vi "MagBrakeToggle (1).vi"(8 "MagBrake Out":bool, 9 "MagBrake In":bool, 10 "MagPressureLimit (PSI)":dbl, 11 "MagBrakeOn?":bool) -> (1 "MagBrake OUTPUT":bool, 2 "MagBrake In":bool, 3 "MagBrakeToggle Complete":bool)   [LabVIEW 2017]
uses:
  Sensors/DataStreamIndex.ctl
  HostDataGLOBAL.vi
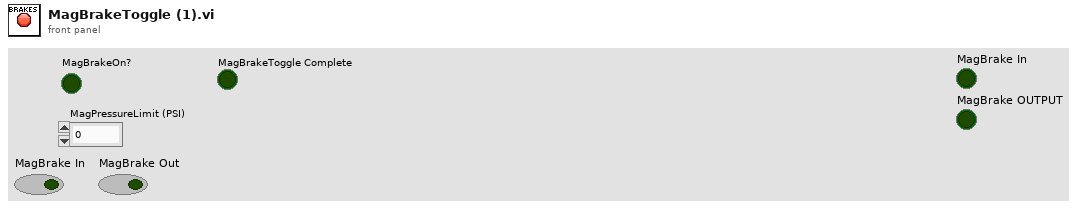
[diagram p1: front panel]
types:
  T1 = typedef "DataStreamIndex.ctl" = enum16{"SuspensionPT (PSI)", "MagBrakePT (PSI)", "Baby HPPT (PSI)", "BigRight HPPT (PSI)", "BigLeft HPPT (PSI)", "HallEffect FrontLeft (V)", "HallEffect FrontRight (V)", "HallEffect BackRight (V)", "HallEffect BackLeft (V)", "LinearPot FrontRight (V)", "LinearPot FrontLeft (V)", "LinearPot BackRight (V)", "LinearPot BackLeft (V)", "Speed (m/s)", "Distance (m)", "Piezo (V)", "Battery Voltage (V)", "Battery Current", "Battery Temperature (C)", "cRIO Temperature (C)", "Right Big Tank Temperature (C)", "Left Big Tank Temperature (C)", "Baby Tank Temperature (C)", "Right Manifold Temperature (C)", "Left Manifold Temperature (C)", "IMU Acceleration (m/s2)", "IMU Pressure (Pa)", "IMU Temperature (C)"}
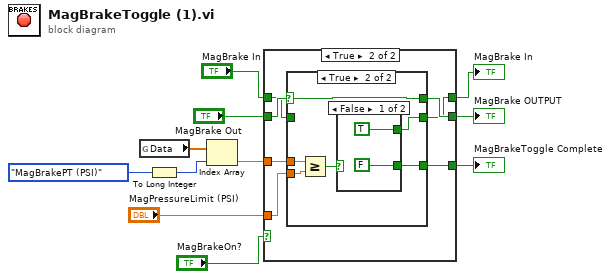
[diagram p0: block diagram]
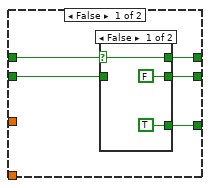
[diagram p2: hidden frame]
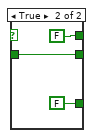
[diagram p3: hidden frame]
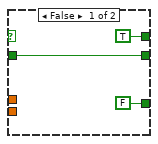
[diagram p4: hidden frame]
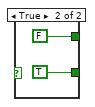
[diagram p5: hidden frame]
diagram:
  n1 = global read "HostDataGLOBAL.vi" "Data"() -> (w4:dbl[])
  n2 = To Long Integer(number=DataStreamIndex."MagBrakePT (PSI)" ("Data Stream Index")) -> (32bit integer=w1:i32)
  n3 = Index Array(array=w4, index=w1) -> (element=w2:dbl)
  n4 = case shown="True" "MagBrakeOn?" {
    tunnel: "MagBrake Out" -> [w13 w29]
    tunnel: [w14 w28] -> w7
    tunnel: [w15 w27] -> w8
    tunnel: "MagBrake In" -> [w16 w26]
    tunnel: "MagPressureLimit (PSI)" -> [_ w25]
    tunnel: w2 -> [_ w24]
    tunnel: [w12 w23] -> w9
    frame False {
      n5 = case shown="False" w16 {
        selector: w16 -> [w18 _]
        tunnel: [w18 FALSE] -> w15
        tunnel: [FALSE ("MagBrake OUTPUT") w21] -> w14
        tunnel: w13 -> [_ w21]
        tunnel: [TRUE FALSE] -> w12
        frame False {
        }
        frame True {
        }
      }
    }
    frame True {
      n6 = case shown="True" w29 {
        selector: w29 -> [_ w38]
        tunnel: [TRUE w38] -> w28
        tunnel: [w31 w36] -> w27
        tunnel: w26 -> [w31 _]
        tunnel: w25 -> [_ w37]
        tunnel: w24 -> [_ w35]
        tunnel: [FALSE w34] -> w23
        frame False {
        }
        frame True {
          n7 = Greater Or Equal?(x=w35, y=w37) -> (x >= y?=w33:bool)
          n8 = case shown="False" w33 {
            tunnel: [TRUE FALSE] -> w36
            tunnel: [FALSE TRUE] -> w34
            frame False {
            }
            frame True {
            }
          }
        }
      }
    }
  }
  "MagBrakeToggle Complete" <- w9
  "MagBrake In" <- w8
  "MagBrake OUTPUT" <- w7
